vi "Taktmerker.vi"(6 "Aktion":enum16{"lesen", "bearbeiten"}(ring), 8 "error in":errorcluster caption="Fehler (Eingang, kein Fehler)") -> (0 "2 s":bool, 1 "1 s":bool, 2 "500 ms":bool, 3 "200 ms":bool, 4 "error out":errorcluster caption="Fehler (Ausgang, kein Fehler)")   [LabVIEW 2020, in "Allgemein.lvlib"]
uses:
  Allgemein.lvlib
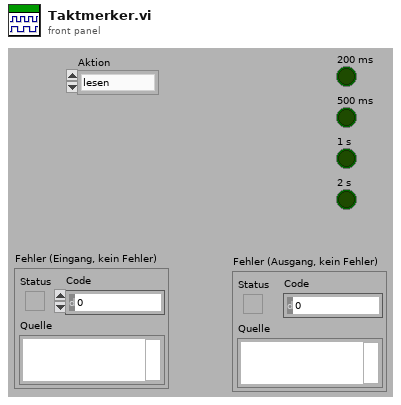
[diagram p1: front panel]
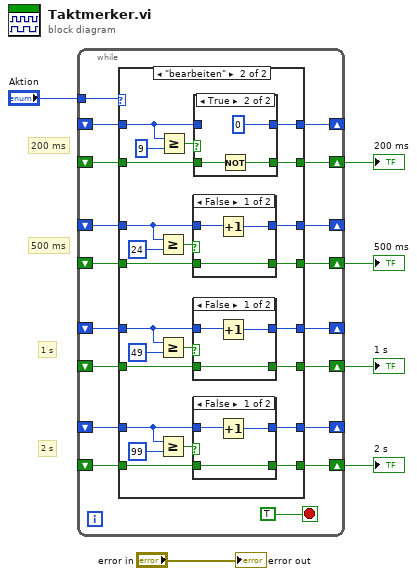
[diagram p0: block diagram]
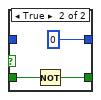
[diagram p3: hidden frame]
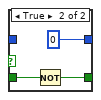
[diagram p4: hidden frame]
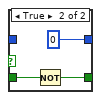
[diagram p5: hidden frame]
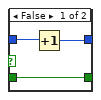
[diagram p6: hidden frame]
diagram:
  # "2 s"
  # "1 s"
  # "500 ms"
  # "200 ms"
  n1 = while {
    shift-right: [w23] -> _
    shift-left: _ -> [w20]
    shift-right: [w22] -> w6
    shift-left: _ -> [w21]
    shift-right: [w16] -> _
    shift-left: _ -> [w19]
    shift-right: [w17] -> w5
    shift-left: _ -> [w18]
    shift-right: [w15] -> _
    shift-left: _ -> [w12]
    shift-right: [w14] -> w4
    shift-left: _ -> [w13]
    shift-right: [w8] -> _
    shift-left: _ -> [w11]
    shift-right: [w9] -> w3
    shift-left: _ -> [w10]
    tunnel: "Aktion" -> [w7]
    stop <- TRUE stop-if-true
    n2 = case shown="\"bearbeiten\"" w7 {
      tunnel: [w32 w56] -> w23
      tunnel: [w31 w55] -> w22
      tunnel: w21 -> [w31 w54]
      tunnel: w20 -> [w32 w52]
      tunnel: w19 -> [w30 w49]
      tunnel: w18 -> [w29 w47]
      tunnel: [w29 w46] -> w17
      tunnel: [w30 w45] -> w16
      tunnel: [w28 w44] -> w15
      tunnel: [w27 w43] -> w14
      tunnel: w13 -> [w27 w42]
      tunnel: w12 -> [w28 w40]
      tunnel: w11 -> [w26 w37]
      tunnel: w10 -> [w25 w35]
      tunnel: [w25 w34] -> w9
      tunnel: [w26 w33] -> w8
      frame "lesen", Default {
      }
      frame "bearbeiten" {
        n3 = Greater Or Equal?(x=w49, y=u8 24) -> (x >= y?=w48:bool)
        n4 = Greater Or Equal?(x=w40, y=u8 49) -> (x >= y?=w41:bool)
        n5 = Greater Or Equal?(x=w37, y=u8 99) -> (x >= y?=w36:bool)
        n6 = Greater Or Equal?(x=w52, y=u8 9) -> (x >= y?=w53:bool)
        n7 = case shown="False" w48 {
          tunnel: [w70 u8 0 ("x+1")] -> w45
          tunnel: w49 -> [w71 _]
          tunnel: [w69 w73] -> w46
          tunnel: w47 -> [w69 w72]
          frame False {
            n8 = Increment(x=w71) -> (x+1=w70:u8)
          }
          frame True {
            n9 = Not(x=w72) -> (.not. x?=w73:bool)
          }
        }
        n10 = case shown="False" w41 {
          tunnel: [w64 u8 0 ("x+1")] -> w44
          tunnel: w40 -> [w65 _]
          tunnel: [w63 w67] -> w43
          tunnel: w42 -> [w63 w66]
          frame False {
            n11 = Increment(x=w65) -> (x+1=w64:u8)
          }
          frame True {
            n12 = Not(x=w66) -> (.not. x?=w67:bool)
          }
        }
        n13 = case shown="False" w36 {
          tunnel: [w58 u8 0 ("x+1")] -> w33
          tunnel: w37 -> [w59 _]
          tunnel: [w57 w61] -> w34
          tunnel: w35 -> [w57 w60]
          frame False {
            n14 = Increment(x=w59) -> (x+1=w58:u8)
          }
          frame True {
            n15 = Not(x=w60) -> (.not. x?=w61:bool)
          }
        }
        n16 = case shown="True" w53 {
          tunnel: [w76 u8 0 ("x+1")] -> w56
          tunnel: w52 -> [w77 _]
          tunnel: [w75 w79] -> w55
          tunnel: w54 -> [w75 w78]
          frame False {
            n17 = Increment(x=w77) -> (x+1=w76:u8)
          }
          frame True {
            n18 = Not(x=w78) -> (.not. x?=w79:bool)
          }
        }
      }
    }
  }
  "200 ms" <- w6
  "500 ms" <- w5
  "1 s" <- w4
  "2 s" <- w3
  "error out" <- "error in"
